vi "Write Alias.vi"(8 "error in":errorcluster, 10 "Alias":string, 11 "Plugin_Channels in":refnum<class "Plugin_Channels.lvclass">) -> (0 "error out":errorcluster, 3 "Plugin_Channels out":refnum<class "Plugin_Channels.lvclass">)   [LabVIEW 2020, in "Plugin.lvlib" / "Plugin_Channels.lvclass"]
doc: "Writes the alias name"
uses:
  Plugin_Channels.lvclass
  Plugin_Channels.lvclass/Plugin_Channels.ctl
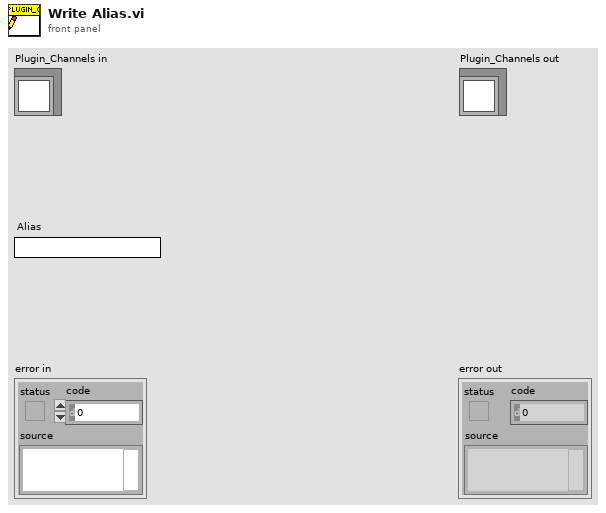
[diagram p1: front panel]
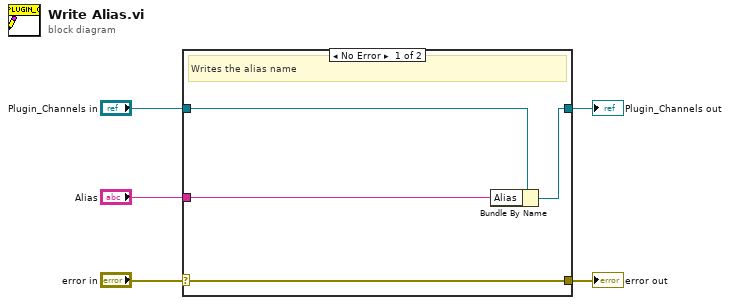
[diagram p0: block diagram]
diagram:
  n1 = case shown="No Error" "error in" {
    selector: "error in" -> [w9 w10]
    tunnel: [w9 w10] -> w4
    tunnel: [w7 w11] -> w2
    tunnel: "Plugin_Channels in" -> [w8 w11]
    tunnel: "Alias" -> [w6 _]
    frame No Error {
      # "Writes the alias name"
      n2 = Bundle By Name(cluster=w8, "Alias"=w6) -> (w7:refnum<class "Plugin_Channels.lvclass">)
    }
    frame Error {
      # "Error"
    }
  }
  "error out" <- w4
  "Plugin_Channels out" <- w2
